vi "Control Mode Read Single.vi"(8 "error in":errorcluster, 9 "Channel Index":i32, 11 "Power Supply In":refnum<class "Power Supply.lvclass">) -> (0 "error out":errorcluster, 1 "Changed or First Call?":bool, 2 "Control Mode CTL":u16, 3 "Power Supply Out":refnum<class "Power Supply.lvclass">)   [LabVIEW 2023, in "Power Supply.lvclass"]
uses:
  Power Supply.lvclass
  Power Supply.lvclass/Power Supply.ctl
  Low Level Capabilities/Control Mode/Control Mode.lvclass
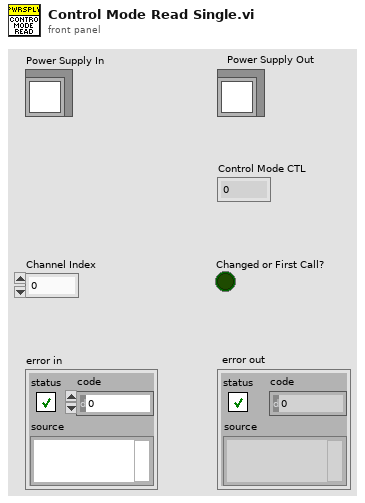
[diagram p1: front panel]
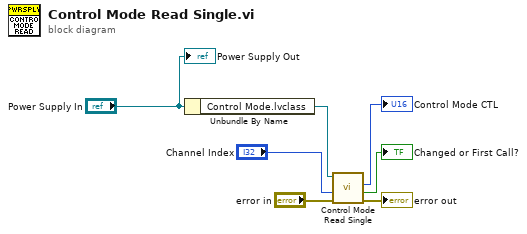
[diagram p0: block diagram]
diagram:
  n1 = Unbundle By Name("Power Supply In") -> ("Control Mode.lvclass"=w1:refnum<class "Control Mode.lvclass">)
  n2 = call-dynamic "Control Mode Read Single.vi"("error in"="error in", "Channel Index"="Channel Index", "Control Mode in"=w1) -> ("error out"=→"error out":errorcluster, "Changed or First Call?"=→"Changed or First Call?":bool, "Control Mode CTL"=→"Control Mode CTL":u16)  [unwired: 5 in, 1 out]
  "Power Supply Out" <- "Power Supply In"
